vi "Create Task.vi"(8 "error in":errorcluster, 10 "Task name":string="WaveformOutputTask", 11 "NI Waveform Output in":refnum<class "NI Waveform Output.lvclass">) -> (0 "error out":errorcluster, 3 "NI Waveform Output out":refnum<class "NI Waveform Output.lvclass">)   [LabVIEW 2023, in "HardwareAbstractionLayer_LVOOP.lvlib" / "NI Waveform Output.lvclass"]
doc: "This VI DAQmx Create Auto Task"
uses:
  NI Waveform Output.lvclass
  NI Waveform Output.lvclass/NI Waveform Output.ctl
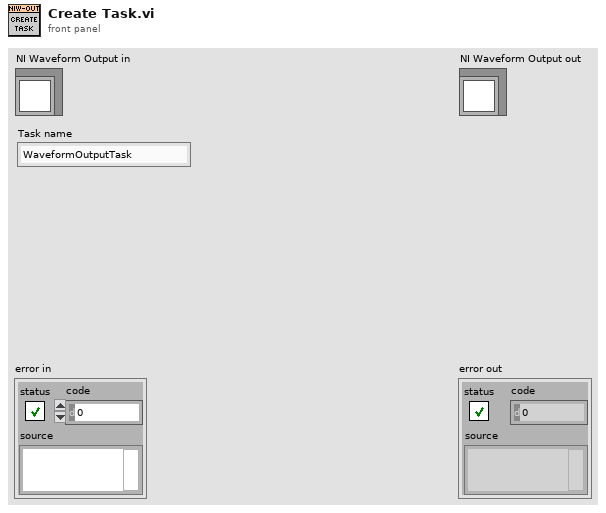
[diagram p1: front panel]
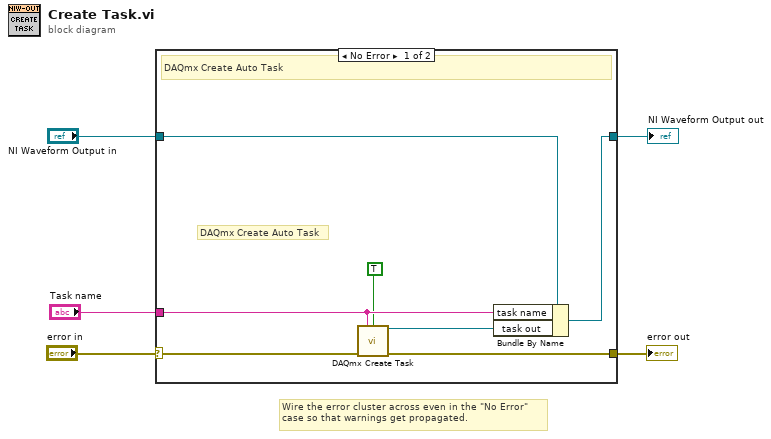
[diagram p0: block diagram]
diagram:
  # "Wire the error cluster across even in the \"No Error\"\ncase so that warnings get propagated."
  n1 = case shown="No Error" "error in" {
    selector: "error in" -> [w12 w14]
    tunnel: [w11 w14] -> w4
    tunnel: [w9 w13] -> w2
    tunnel: "NI Waveform Output in" -> [w10 w13]
    tunnel: "Task name" -> [w7 _]
    frame No Error {
      # "DAQmx Create Auto Task"
      # "DAQmx Create Auto Task"
      n2 = call <vilib>:"DAQmx Create Task.vi"("new task name"=w7, "auto cleanup"=TRUE, "error in"=w12) -> ("task out"=w8:refnum<k21>, "error out"=w11:errorcluster)  [unwired: 11 in]
      n3 = Bundle By Name(cluster=w10, "task name"=w7, "task out"=w8) -> (w9:refnum<class "NI Waveform Output.lvclass">)
    }
    frame Error {
    }
  }
  "error out" <- w4
  "NI Waveform Output out" <- w2
